vi "GUI_HPD_CCD.vi"() -> ()   [LabVIEW 2013]
uses:
  shared programs/GUI_Template/GUI_master/tcp_new_data_event.ctl
  shared programs/GUI_Template/GUI_master/tcp new data cluster.ctl
  <vilib>/vision/Image Controls.llb/IMAQ Image.ctl
panel:
  out "image::3":T1(plugin-control) caption="image"
  out "GUIdevice 3":string="HPD_CCD"
  in  "exposure::2":dbl=0.001 caption="exposure" min=0.0001 max=1.0 format="%_4p"
  in  "GUIdevice 2":string="HPD_CCD"
  out "image::2":T1(plugin-control) caption="image"
  out "tcp data event":T2
  in  "Refresh Button":bool
  in  "Select device":string(combo)="FrogHPD"
  in  "stop":bool
  in  "trigger::1":bool caption="Trigger"
  in  "gain::1":dbl=0.001 caption="gain" min=0.0 max=24.0 format="%_4f"
  in  "centroidy::1":dbl=0.001 caption="centroid y" min=0.0 max=0.0 format="%_4f"
  in  "centroidx::1":dbl=0.001 caption="centroid x" min=0.0 max=0.0 format="%_4f"
  in  "exposure::1":dbl=0.001 caption="exposure" min=0.0001 max=1.0 format="%_4p"
  out "image::1":T1(plugin-control) caption="image"
  out "GUIdevice 1":string="HPD_CCD"
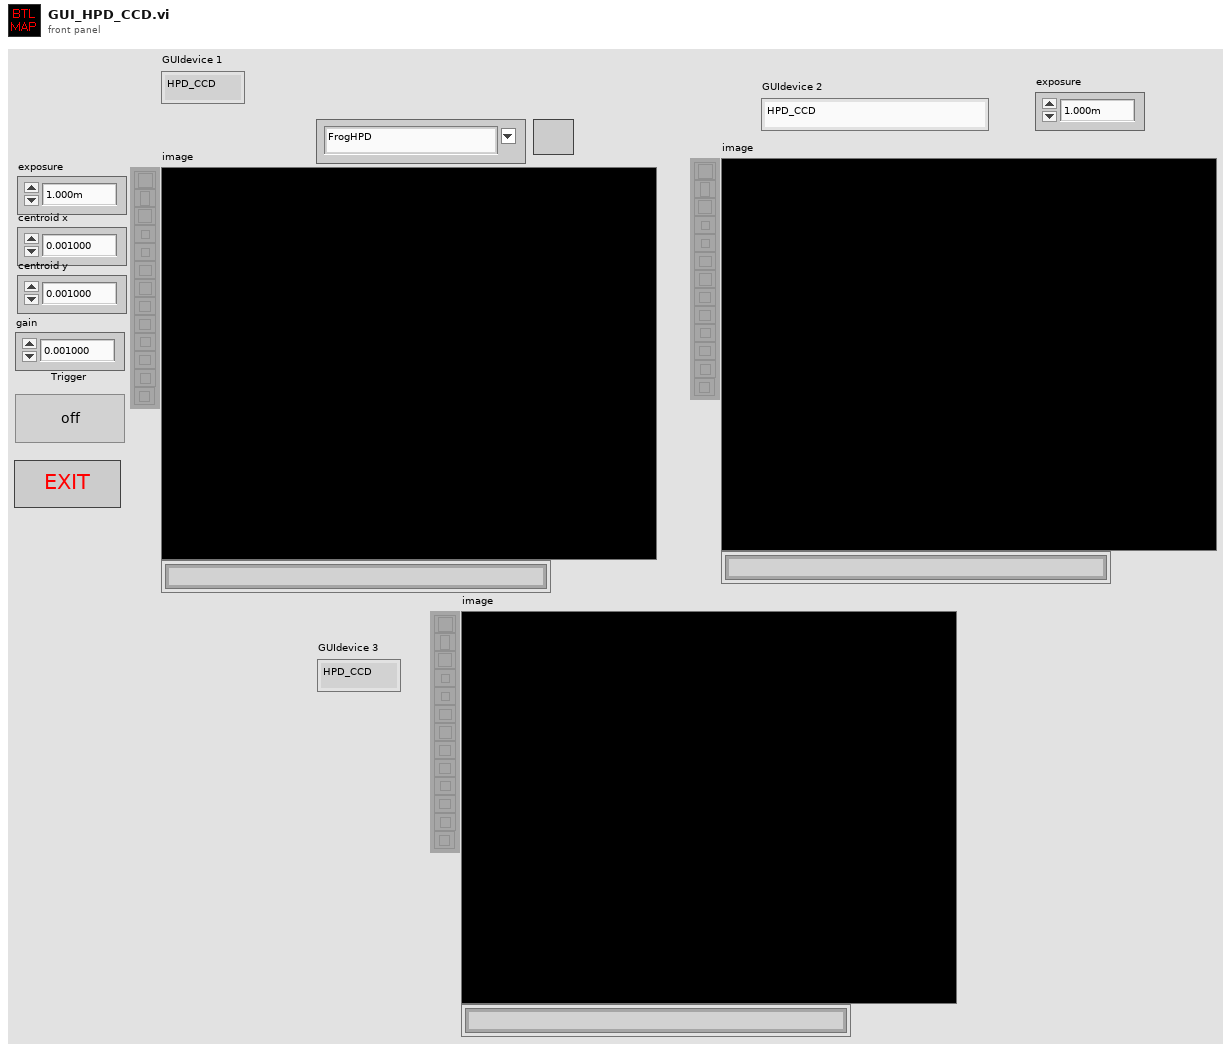
[diagram p1: front panel]
types:
  T1 = typedef "IMAQ Image.ctl" = refnum<image>
  T2 = typedef "tcp_new_data_event.ctl" = refnum<user-event>
  T3 = enum32{"invalid app kind", "Development System", "Run Time System", "Student Edition", "Embedded LabVIEW", "Evaluation", "Custom"}
  T4 = typedef "tcp new data cluster.ctl" = cluster{"EventEnum":enum16{"new data", "connection status update"}, "Device name":string}
  T5 = enum32{"Invalid", "Standard", "Closed", "Hidden", "Minimized", "Maximized"}
  T6 = cluster{"Core":cluster{"Current VI Reference":refnum<vi>, "Close Panel on Exit?":bool}, "Your Boolean data":bool, "Your string data":string, "SuperGUI":cluster{"STOP queue":refnum<queue>, "SuperGUI ref":refnum<vi>}}
  T7 = cluster{"STOP queue":refnum<queue>, "SuperGUI ref":refnum<vi>}
  T8 = cluster{"Current VI Reference":refnum<vi>, "Close Panel on Exit?":bool}
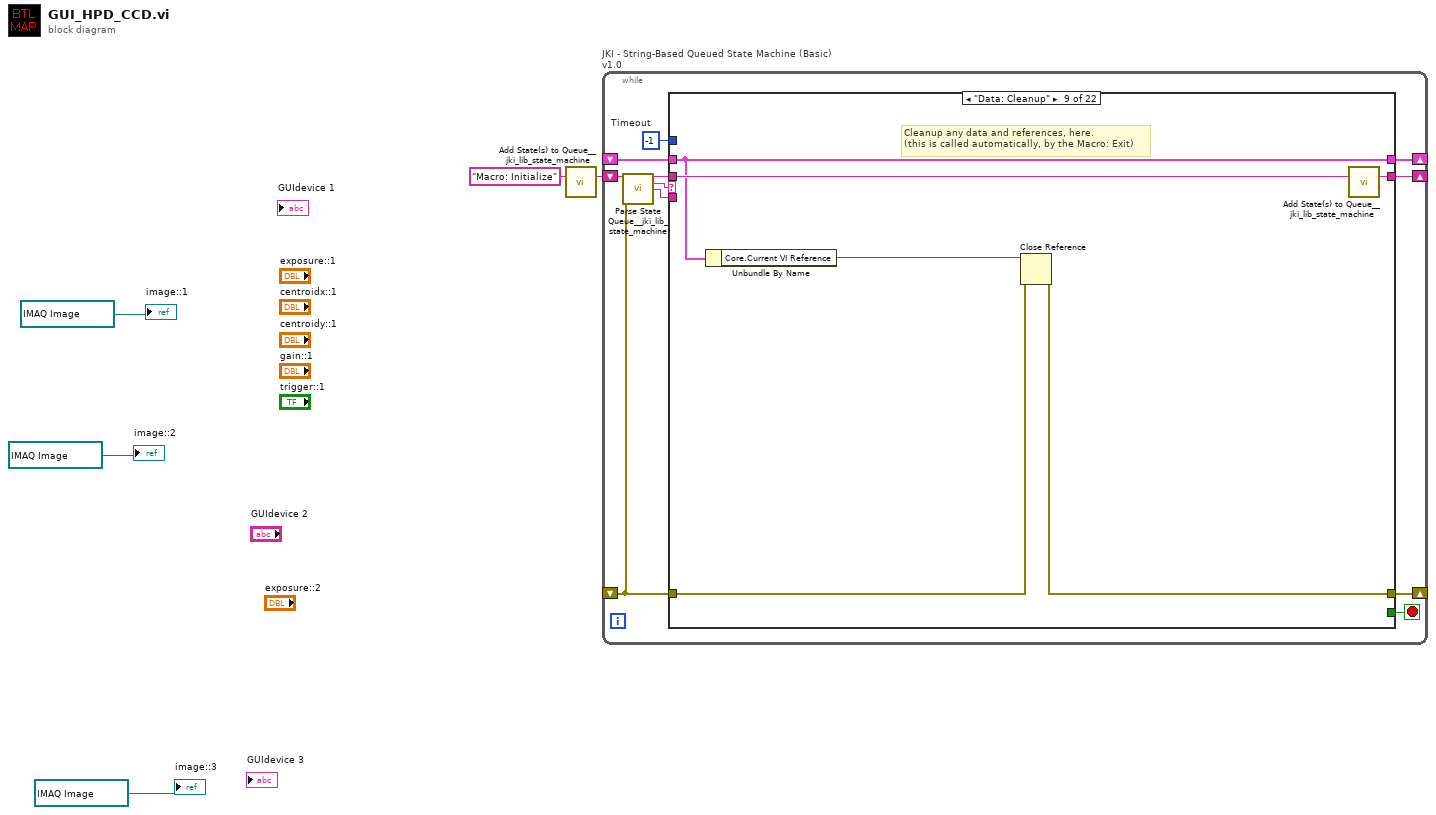
[diagram p0: block diagram]
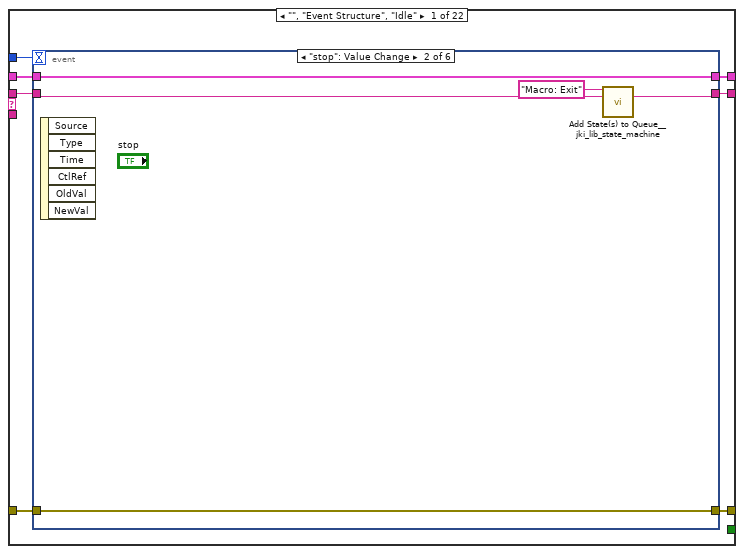
[diagram p2: hidden frame]
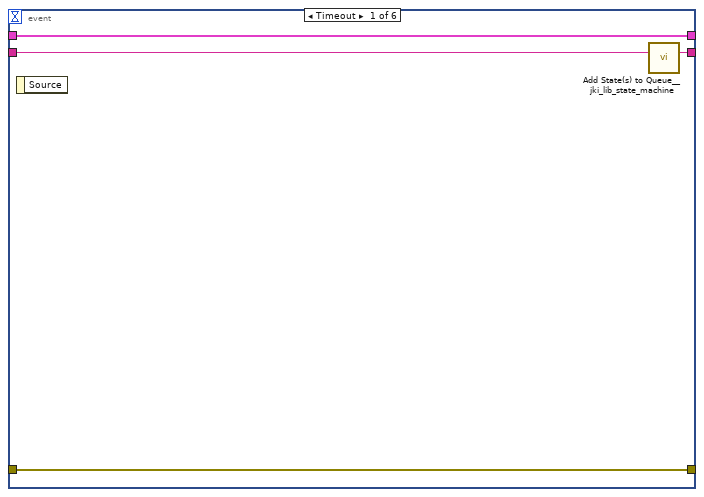
[diagram p3: hidden frame]
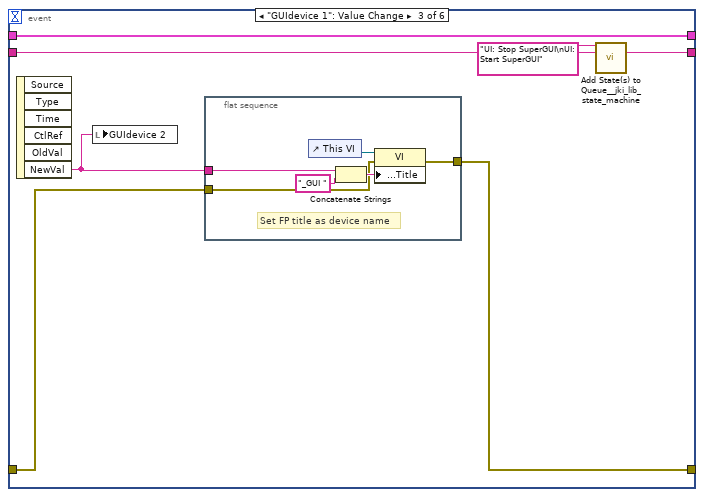
[diagram p4: hidden frame]
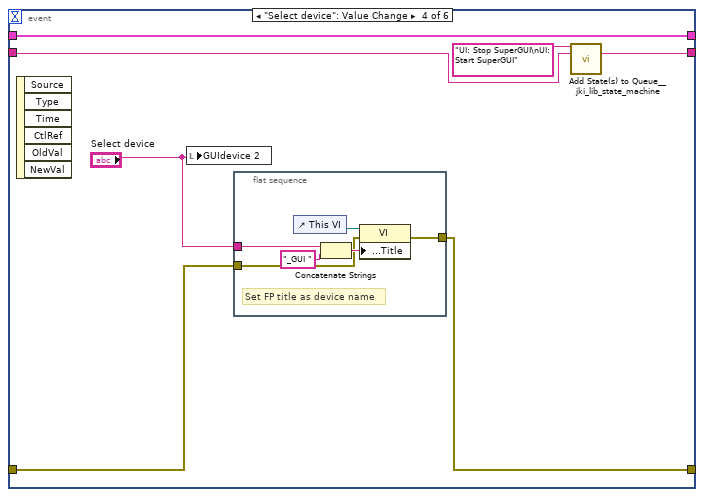
[diagram p5: hidden frame]
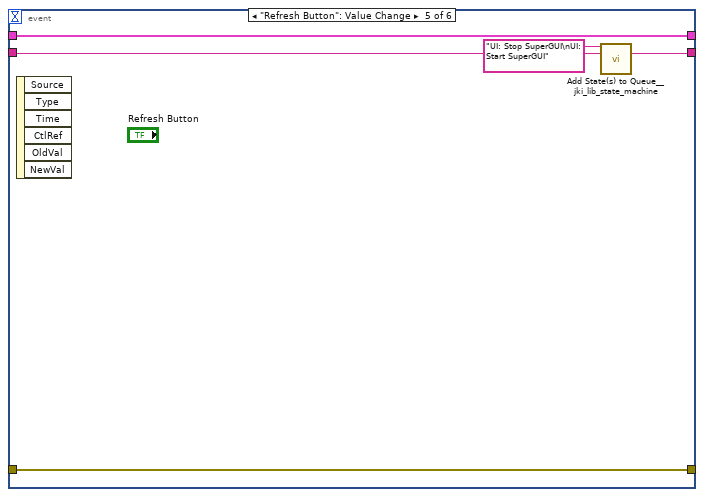
[diagram p6: hidden frame]
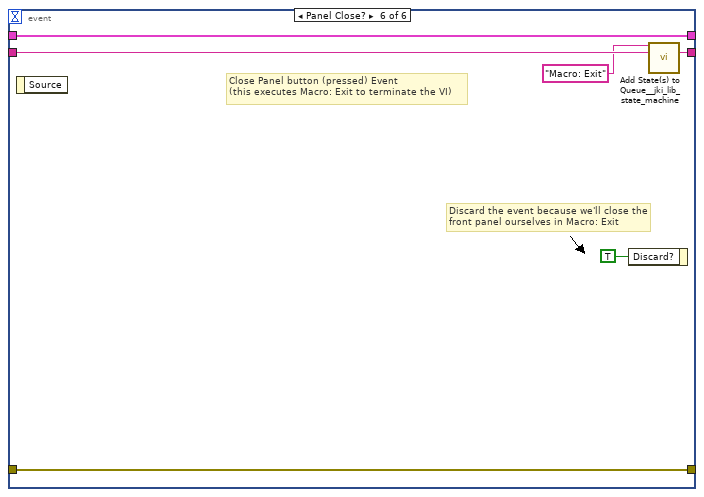
[diagram p7: hidden frame]
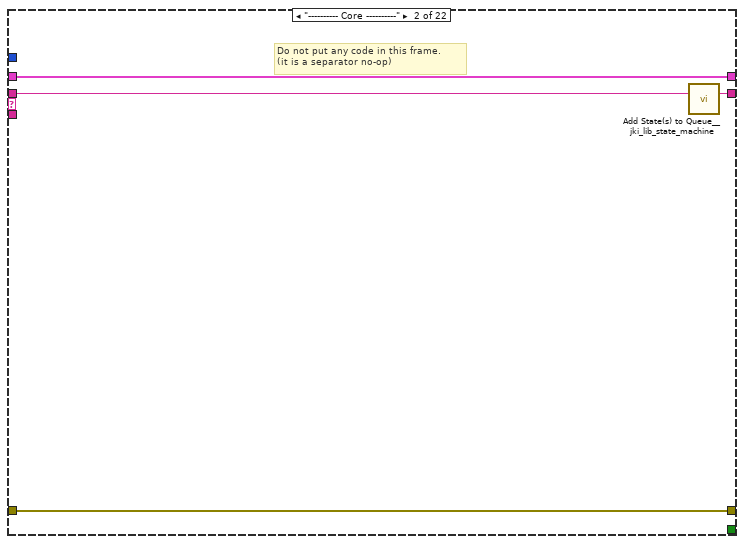
[diagram p8: hidden frame]
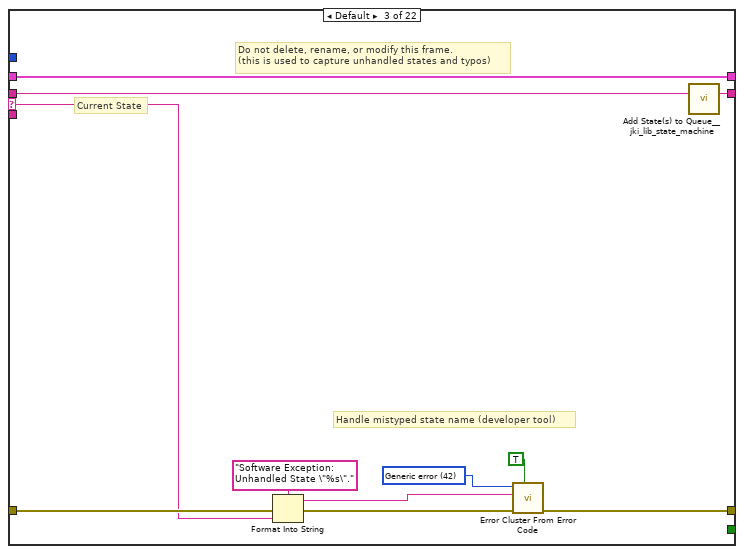
[diagram p9: hidden frame]
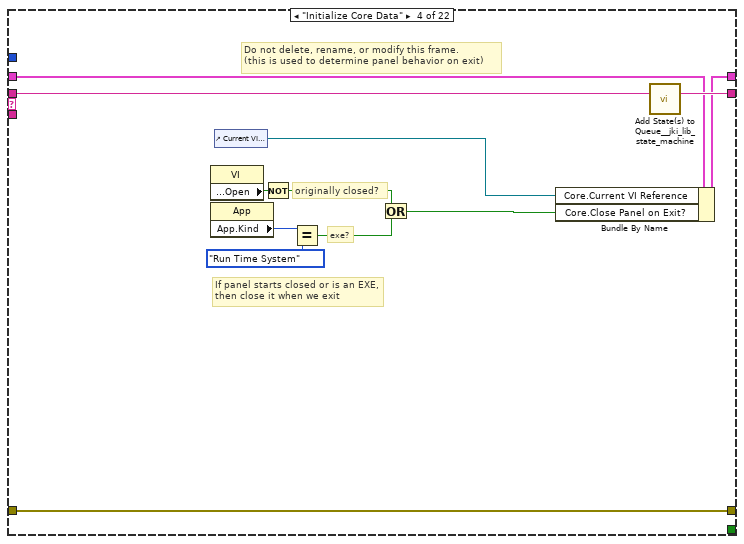
[diagram p10: hidden frame]
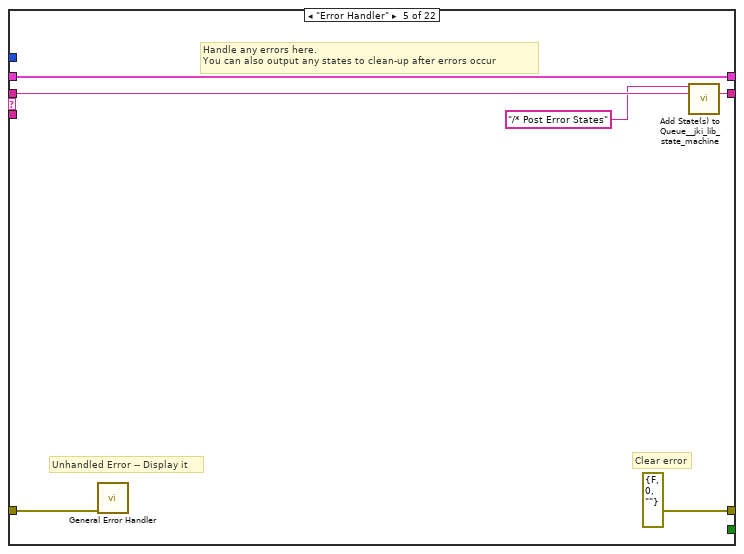
[diagram p11: hidden frame]
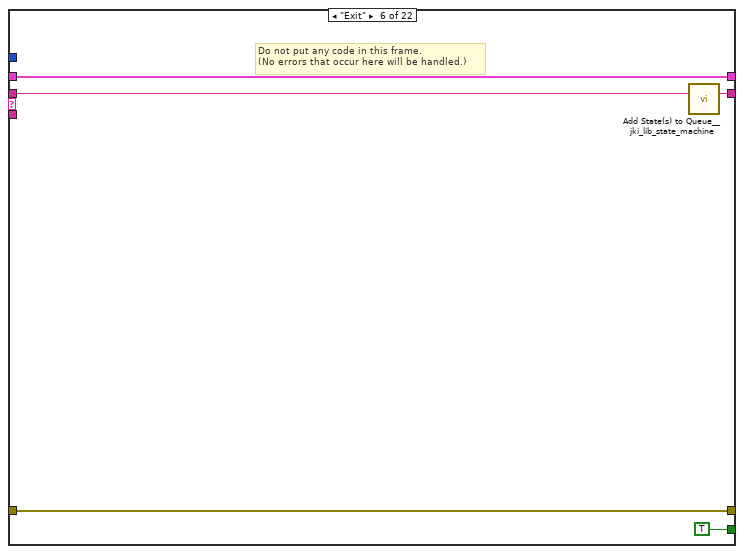
[diagram p12: hidden frame]
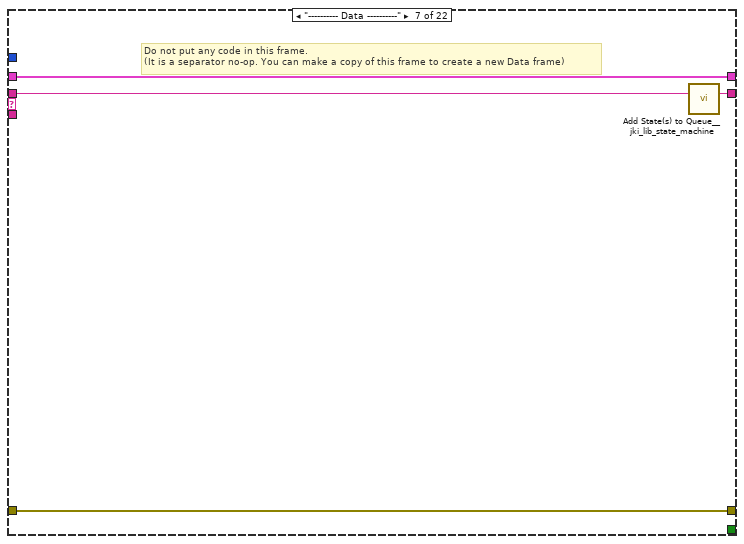
[diagram p13: hidden frame]
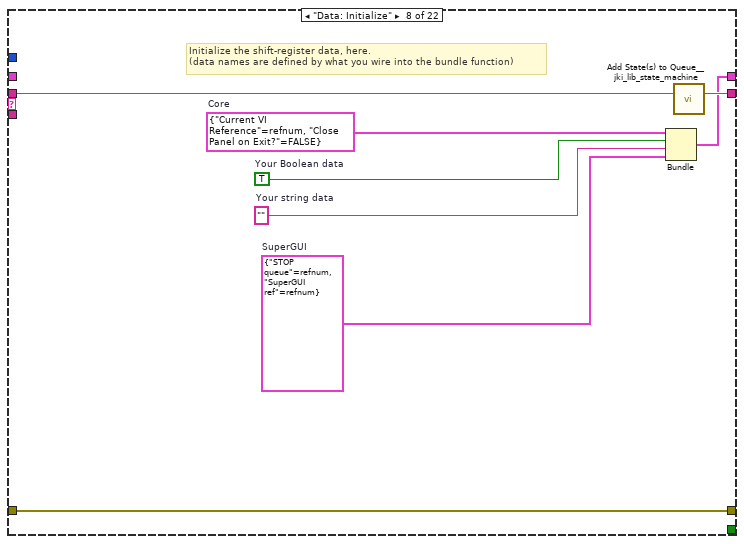
[diagram p14: hidden frame]
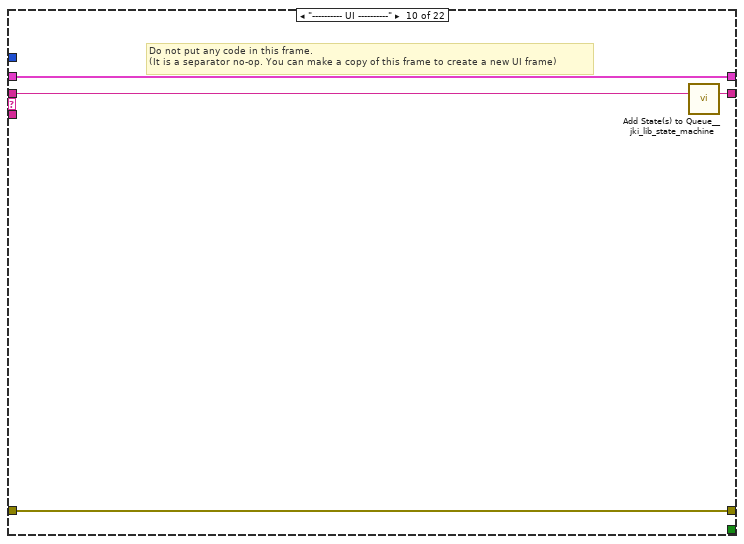
[diagram p15: hidden frame]
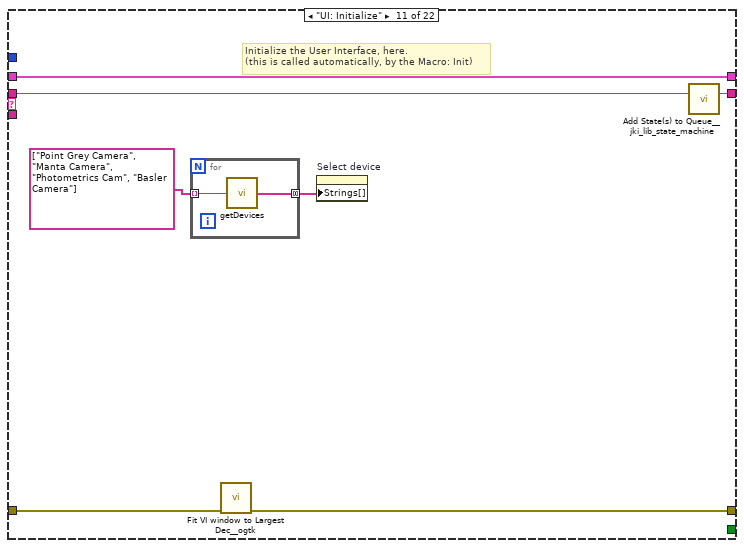
[diagram p16: hidden frame]
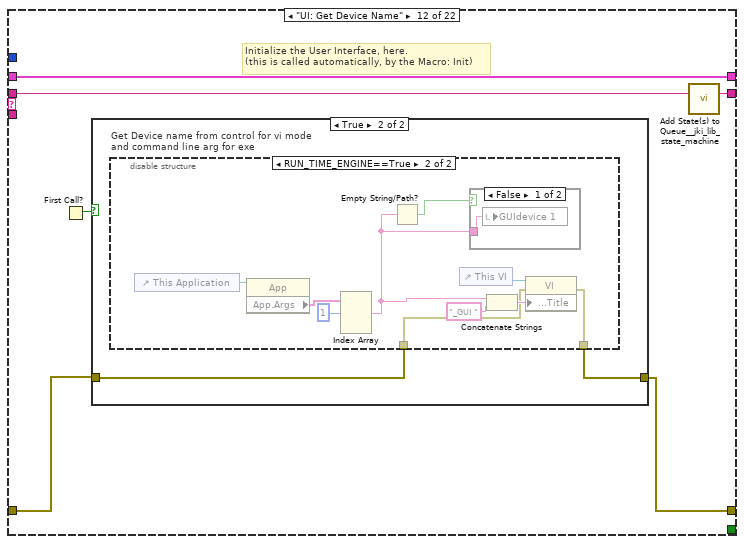
[diagram p17: hidden frame]
diagram:
  n1 = call <vilib>:"Add State(s) to Queue__jki_lib_state_machine.vi"("State(s) in (\"\")"="Macro: Initialize") -> ("States Out"=w4:string)  [unwired: 14 in]
  n2 = while "JKI - String-Based Queued State Machine (Basic) v1.0" {
    shift-right: [w9] -> _
    shift-left: _ -> [w8]
    shift-right: [w12] -> _
    shift-left: _ -> [w6]
    shift-right: [w11] -> _
    shift-left: w4 -> [w13]
    stop <- w10 stop-if-true
    w7 = -1  # Timeout
    n3 = call <vilib>:"Parse State Queue__jki_lib_state_machine.vi"("State Queue"=w13, "Error In (no error)"=w6) -> ("Remaining States"=w15:string, "Current State"=w16:string, "Arguments"=w14:string)  [unwired: 11 in]
    n4 = case shown="\"Data: Cleanup\"" w16 {
      selector: w16 -> [_ _ w74 _ _ _ _ _ _ _ _ _ _ _ _ _ _ _ _ _ _ _]
      tunnel: w15 -> [w23 w73 w78 w96 w102 w107 w111 w119 w125 w129 w136 w144 w179 w187 w193 w204 w230 w235 w245 w249 w253 w257]
      tunnel: w14 -> [_ _ _ _ _ _ _ _ _ _ _ _ _ _ w188 w198 _ _ _ _ _ _]
      tunnel: w8 -> [w21 w70 w76 w87 w99 w105 w108 _ w120 w126 w134 w142 w170 w182 w191 w200 w227 w232 w242 w246 w250 w254]
      tunnel: [w20 w71 w80 w93 errorcluster {"status"=FALSE, "code"=0, "source"=""} ("error out") w104 w109 w116 w121 w127 w132 w139 w163 w180 w189 w201 w228 w233 w243 w247 w251 w255] -> w12
      tunnel: w6 -> [w19 w71 w79 w93 w98 w104 w109 w116 w122 w127 w133 w140 w164 w181 w190 w202 w228 w233 w243 w247 w251 w255]
      tunnel: [w22 w72 w77 w95 w101 w106 w110 w118 w124 w128 w135 w143 w178 w186 w192 w203 w229 w234 w244 w248 w252 w256] -> w11
      tunnel: [_ _ _ _ _ TRUE _ _ _ _ _ _ _ _ _ _ _ _ _ _ _ _] -> w10
      tunnel: [w18 w70 w76 w94 w99 w105 w108 w117 w120 w126 w134 w142 w169 w182 w191 w200 w227 w232 w242 w246 w250 w254] -> w9
      tunnel: w7 -> [w17 _ _ _ _ _ _ _ _ _ _ _ _ _ _ _ _ _ _ _ _ _]
      frame "", "Event Structure", "Idle" {
        n5 = event shown="[1] \"stop\": Value Change" {
          selector: _ -> [_ _ _ _ _ _]
          dyn-events: _ -> [_ _ _ _ _ _]
          timeout: w17 -> [_ _ _ _ _ _]
          tunnel: w23 -> [w27 w30 w36 w48 w61 w69]
          tunnel: [w26 w29 w35 w47 w60 w68] -> w22
          tunnel: w21 -> [w24 w32 w39 w52 w63 w66]
          tunnel: [w25 w31 w37 w50 w62 w67] -> w20
          tunnel: w19 -> [w25 w31 w38 w51 w62 w67]
          tunnel: [w24 w32 w39 w52 w63 w66] -> w18
          event Timeout {
            n6 = event-data() -> ()  [unwired: 1 in, 1 out]
            n7 = call <vilib>:"Add State(s) to Queue__jki_lib_state_machine.vi"("State(s) in (\"\")"=w27) -> ("States Out"=w26:string)  [unwired: 14 in]
          }
          event "stop": Value Change {
            n8 = event-data() -> ()  [unwired: 1 in, 6 out]
            n9 = call <vilib>:"Add State(s) to Queue__jki_lib_state_machine.vi"("State(s) in Front (\"\")"="Macro: Exit", "State(s) in (\"\")"=w30) -> ("States Out"=w29:string)  [unwired: 13 in]
          }
          event "GUIdevice 1": Value Change {
            n10 = event-data() -> ("NewVal"=w33:string)  [unwired: 1 in, 5 out]
            n11 = local write "GUIdevice 2"(w33) -> ()
            n12 = flat-sequence {
              tunnel: [w42] -> w37
              tunnel: w38 -> [w41]
              tunnel: w33 -> [w40]
              frame #0 {
                # "Set FP title as device name"
                n13 = control-ref of="This VI"() -> (w45:refnum<vi>)
                n14 = Concatenate Strings(w40, "_GUI ") -> (w44:string)
                n15 = property class="VI"(reference=w45, error in=w41, "Front Panel.Title"=w44) -> (error out=w42:errorcluster)  [unwired: 1 out]
              }
            }
            n16 = call <vilib>:"Add State(s) to Queue__jki_lib_state_machine.vi"("State(s) in Front (\"\")"="UI: Stop SuperGUI\nUI: Start SuperGUI", "State(s) in (\"\")"=w36) -> ("States Out"=w35:string)  [unwired: 13 in]
          }
          event "Select device": Value Change {
            n17 = event-data() -> ()  [unwired: 1 in, 6 out]
            n18 = local write "GUIdevice 2"("Select device") -> ()
            n19 = flat-sequence {
              tunnel: [w55] -> w50
              tunnel: w51 -> [w54]
              tunnel: "Select device" -> [w53]
              frame #0 {
                # "Set FP title as device name"
                n20 = control-ref of="This VI"() -> (w58:refnum<vi>)
                n21 = Concatenate Strings(w53, "_GUI ") -> (w57:string)
                n22 = property class="VI"(reference=w58, error in=w54, "Front Panel.Title"=w57) -> (error out=w55:errorcluster)  [unwired: 1 out]
              }
            }
            n23 = call <vilib>:"Add State(s) to Queue__jki_lib_state_machine.vi"("State(s) in Front (\"\")"="UI: Stop SuperGUI\nUI: Start SuperGUI", "State(s) in (\"\")"=w48) -> ("States Out"=w47:string)  [unwired: 13 in]
          }
          event "Refresh Button": Value Change {
            n24 = event-data() -> ()  [unwired: 1 in, 6 out]
            n25 = call <vilib>:"Add State(s) to Queue__jki_lib_state_machine.vi"("State(s) in Front (\"\")"="UI: Stop SuperGUI\nUI: Start SuperGUI", "State(s) in (\"\")"=w61) -> ("States Out"=w60:string)  [unwired: 13 in]
          }
          event Panel Close? {
            # "Discard the event because we'll close the front panel ourselves in Macro: Exit"
            # "Close Panel button (pressed) Event\n(this executes Macro: Exit to terminate the VI)"
            n26 = event-data() -> ()  [unwired: 1 in, 1 out]
            n27 = event-data("Discard?"=TRUE) -> ()  [unwired: 1 in, 1 out]
            n28 = call <vilib>:"Add State(s) to Queue__jki_lib_state_machine.vi"("State(s) in Front (\"\")"="Macro: Exit", "State(s) in (\"\")"=w69) -> ("States Out"=w68:string)  [unwired: 13 in]
          }
        }
      }
      frame "---------- Core ----------" {
        # "Do not put any code in this frame.\n(it is a separator no-op)"
        n29 = call <vilib>:"Add State(s) to Queue__jki_lib_state_machine.vi"("State(s) in (\"\")"=w73) -> ("States Out"=w72:string)  [unwired: 14 in]
      }
      frame Default {
        w83 = 42 items=["No error", "Argument error", "Memory is full", "Out of zone", "End of file", "File already open", "Generic file I/O error", "File not found", "File permission error", "Disk is full", "Duplicate path", "Too many files open", "System feature not enabled", "Resource file not found", "Cannot add resource", "Resource not found", "Image not found", "Image memory error", "Pen does not exist", "Config type invalid", "Config token not found", "Config parse error", "Config memory error", "Bad external code format", "Bad external code offset", "External code not present", "Null window", "Destroy window error", "Null menu", "Print aborted", "Bad print record", "Print driver error", "Windows error during printing", "Memory error during printing", "Print dialog error", "Generic print error", "Invalid device refnum", "Device not found", "Device parameter error", "Device unit error", "Cannot open device", "Device call aborted", "Generic error", "Cancelled by user", "Object ID too low", "Object ID too high", "Object not in heap", "Unknown heap", "Unknown object (invalid DefProc)", "Unknown object (DefProc not in table)", "Message out of range", "Invalid (null) method", "Unknown message", "Manager call not supported", "Bad address", "Network operation in progress", "Network operation timed out", "Connection is busy", "Network attribute not supported", "Network error", "Address in use", "System out of memory", "Connection aborted", "Connection refused", "Not connected", "Already connected", "Connection closed", "Initialization error (interapplication manager)", "Bad occurrence", "Wait on unbound occurrence handler", "Occurrence queue overflow", "Datalog type conflict", "Unused", "Unrecognized type (interapplication manager)", "Memory corrupt", "Failed to make temporary DLL", "Old CIN version", "Drag socket not found", "Failed to load drop-object", "Failed to register OLE object", "Failed to release OLE object", "Format specifier type mismatch", "Unknown format specifier", "Too few format specifiers", "Too many format specifiers", "Scan failed", "Newer CIN version", "Error converting to variant", "Runtime menu error", "Password tampered", "Variant attribute not found", "Incompatible variant data type", "Event data is not available", "Event Store is not present", "Occurrence is not found", "Event Queue is not created", "Event info is not available", "Refnum passed is NULL", "Error retrieving Class GUID", "Error retrieving CoClass GUID", "Error retrieving TypeLib GUID.", "Bad built application magic bytes.", "Specific driver is different from the specific driver associated with the Logical Name.", "There is no session opened to the class driver.", "Max Error", "MAX - Error with config objects", "MAX - Error loading configuration", "MAX - Group not supported"]
        # "Current State"
        # "Do not delete, rename, or modify this frame.\n(this is used to capture unhandled states and typos)"
        # "Handle mistyped state name (developer tool)"
        n30 = Format Into String(format string="Software Exception: Unhandled State \"%s\"." ("message"), error in=w79, w74) -> (resulting string=w82:string, error out=w81:errorcluster)  [unwired: 1 in]
        n31 = call <vilib>:"Error Cluster From Error Code.vi"("show call chain? (False)"=TRUE, "error in (no error)"=w81, "error message (\"\")"=w82, "error code (0)"=w83) -> ("error out"=w80:errorcluster)  [unwired: 5 in]
        n32 = call <vilib>:"Add State(s) to Queue__jki_lib_state_machine.vi"("State(s) in (\"\")"=w78) -> ("States Out"=w77:string)  [unwired: 14 in]
      }
      frame "Initialize Core Data" {
        # "Do not delete, rename, or modify this frame.\n(this is used to determine panel behavior on exit)"
        # "originally closed?"
        # "exe?"
        # "If panel starts closed or is an EXE, then close it when we exit"
        n33 = property class="VI"() -> ("Front Panel.Open"=w92:bool)  [unwired: 2 in, 2 out]
        n34 = property class="App"() -> ("App.Kind"=w91:T3)  [unwired: 2 in, 2 out]
        n35 = control-ref of="Current VI Reference"() -> (w85:refnum<vi>)
        n36 = Not(x=w92) -> (.not. x?=w89:bool)
        n37 = Equal?(x=w91, y=T3."Run Time System" ("Application:Kind")) -> (x = y?=w88:bool)
        n38 = Or(x=w89, y=w88) -> (x .or. y?=w86:bool)
        n39 = Bundle By Name(cluster=w87, "Core.Current VI Reference"=w85, "Core.Close Panel on Exit?"=w86) -> (w94:T6)
        n40 = call <vilib>:"Add State(s) to Queue__jki_lib_state_machine.vi"("State(s) in (\"\")"=w96) -> ("States Out"=w95:string)  [unwired: 14 in]
      }
      frame "Error Handler" {
        # "Unhandled Error -- Display it"
        # "Handle any errors here.\nYou can also output any states to clean-up after errors occur"
        # "Clear error"
        n41 = call <vilib>:"General Error Handler.vi"("error in (no error)"=w98) -> ()  [unwired: 10 in, 5 out]
        n42 = call <vilib>:"Add State(s) to Queue__jki_lib_state_machine.vi"("State(s) in Front (\"\")"="/* Post Error States", "State(s) in (\"\")"=w102) -> ("States Out"=w101:string)  [unwired: 13 in]
      }
      frame "Exit" {
        # "Do not put any code in this frame.\n(No errors that occur here will be handled.)"
        n43 = call <vilib>:"Add State(s) to Queue__jki_lib_state_machine.vi"("State(s) in (\"\")"=w107) -> ("States Out"=w106:string)  [unwired: 14 in]
      }
      frame "---------- Data ----------" {
        # "Do not put any code in this frame.\n(It is a separator no-op. You can make a copy of this frame to create a new Data frame)"
        n44 = call <vilib>:"Add State(s) to Queue__jki_lib_state_machine.vi"("State(s) in (\"\")"=w111) -> ("States Out"=w110:string)  [unwired: 14 in]
      }
      frame "Data: Initialize" {
        w112 = T7 {"STOP queue"=refnum, "SuperGUI ref"=refnum}  # SuperGUI
        w113 = T8 {"Current VI Reference"=refnum, "Close Panel on Exit?"=FALSE}  # Core
        w115 = TRUE  # Your Boolean data
        w114 = ""  # Your string data
        # "Initialize the shift-register data, here.\n(data names are defined by what you wire into the bundle function)"
        n45 = Bundle("Core"=w113, "Your Boolean data"=w115, "Your string data"=w114, "SuperGUI"=w112) -> (w117:T6)  [unwired: 1 in]
        n46 = call <vilib>:"Add State(s) to Queue__jki_lib_state_machine.vi"("State(s) in (\"\")"=w119) -> ("States Out"=w118:string)  [unwired: 14 in]
      }
      frame "Data: Cleanup" {
        # "Cleanup any data and references, here.\n(this is called automatically, by the Macro: Exit)"
        n47 = Unbundle By Name(w120) -> ("Core.Current VI Reference"=w123:refnum<vi>)
        n48 = Close Reference(reference=w123, error in (no error)=w122) -> (error out=w121:errorcluster)
        n49 = call <vilib>:"Add State(s) to Queue__jki_lib_state_machine.vi"("State(s) in (\"\")"=w125) -> ("States Out"=w124:string)  [unwired: 14 in]
      }
      frame "---------- UI ----------" {
        # "Do not put any code in this frame.\n(It is a separator no-op. You can make a copy of this frame to create a new UI frame)"
        n50 = call <vilib>:"Add State(s) to Queue__jki_lib_state_machine.vi"("State(s) in (\"\")"=w129) -> ("States Out"=w128:string)  [unwired: 14 in]
      }
      frame "UI: Initialize" {
        # "Initialize the User Interface, here.\n(this is called automatically, by the Macro: Init)"
        n51 = for {
          tunnel: string[] ["Point Grey Camera", "Manta Camera", "Photometrics Cam", "Basler Camera"] -> [w138] mode=indexing
          tunnel: [w137] -> w130 mode=concatenating
          n52 = call "getDevices.vi"("Device Class"=w138) -> ("All Devices"=w137:string[])
        }
        n53 = call <userlib>:"Fit VI window to Largest Dec__ogtk.vi"("error in (no error)"=w133) -> ("error out"=w132:errorcluster)  [unwired: 5 in, 1 out]
        n54 = property on="Select device" class="CmbBox"("Strings[]"=w130) -> ()  [unwired: 2 in, 2 out]
        n55 = call <vilib>:"Add State(s) to Queue__jki_lib_state_machine.vi"("State(s) in (\"\")"=w136) -> ("States Out"=w135:string)  [unwired: 14 in]
      }
      frame "UI: Get Device Name" {
        # "Initialize the User Interface, here.\n(this is called automatically, by the Macro: Init)"
        n56 = First Call?() -> (First Call?: T/F=w141:bool)
        n57 = case shown="True" w141 {
          tunnel: w140 -> [w145 w147]
          tunnel: [w145 w146] -> w139
          frame False {
          }
          frame True {
            n58 = disable-structure "Get Device name from control for vi mode\nand command line arg for exe" shown="RUN_TIME_ENGINE==True" {
              disable-tunnel: w147 -> [w148 w150]
              disable-tunnel: [w148 w149] -> w146
              frame condition #0 (active) {
              }
              frame condition #1 {
                n59 = control-ref of="This Application"() -> (w158:refnum<vi>)
                n60 = property class="App"(reference=w158) -> ("App.Args"=w157:string[])  [unwired: 1 in, 2 out]
                n61 = Index Array(array=w157, index #1=1 ("index")) -> (element #1=w151:string)  [unwired: 2 in, 2 out]
                n62 = Empty String/Path?(string/path=w151) -> (empty?=w155:bool)
                n63 = control-ref of="This VI"() -> (w154:refnum<vi>)
                n64 = case shown="False" w155 {
                  tunnel: w151 -> [w159 _]
                  frame False {
                    n65 = local write "GUIdevice 1"(w159) -> ()
                  }
                  frame True {
                  }
                }
                n66 = Concatenate Strings(w151, "_GUI ") -> (w153:string)
                n67 = property class="VI"(reference=w154, error in=w150, "Front Panel.Title"=w153) -> (error out=w149:errorcluster)  [unwired: 1 out]
              }
            }
          }
        }
        n68 = call <vilib>:"Add State(s) to Queue__jki_lib_state_machine.vi"("State(s) in (\"\")"=w144) -> ("States Out"=w143:string)  [unwired: 14 in]
      }
      frame "UI: Start SuperGUI" {
        # "create stop queue for supergui and its clones"
        # "x100 abort will be dependent on caller VI\nx80 abort will be independent of caller vi, this will abort vi when labview is closed."
        # "Start SuperGUI asynchronous way"
        n69 = vi-ref "GUI_Master_subvi_reentrant_queues.vi"() -> (w162:refnum<vi>)
        n70 = property class="VI"(reference=w162) -> ("Path"=w161:path)  [unwired: 1 in, 2 out]
        n71 = Create User Event(user event datatype=T4 {"EventEnum"=enum."new data", "Device name"="Device name"} ("New Event"), error in=w164) -> (user event=w165:refnum<user-event>, error out=w171:errorcluster)
        "tcp data event" <- w165
        n72 = control-ref of="This Application"() -> (w168:refnum<vi>)
        n73 = control-ref of="This VI"() -> (w167:refnum<vi>)
        n74 = Open VI Reference(type specifier VI Refnum (for type only)=refnum<vi> refnum, vi path=w161, options=256) -> (vi reference=w177:refnum<vi>, error out=w176:errorcluster)  [unwired: 3 in]
        n75 = register-events(w165) -> ()  [unwired: 2 in, 2 out]
        n76 = call "supergui create stop queue.vi"() -> ("STOP Queue out"=w173:refnum<queue>)  [unwired: 11 in]
        n77 = Current VI's Menubar() -> (w166:refnum<k9>)
        n78 = call-by-ref "Start Asynchronous Call"(reference=w177, error in=w176, "STOP Queue in"=w173, "This Application"=w168, 8:"error in (no error)"=w171, "tcp data event"=w165, "Caller menu reference"=w166, "Caller VI ref"=w167) -> (reference out=w160:refnum<vi>, error out=w163:errorcluster)  [unwired: 5 in, 1 out]
        n79 = Bundle By Name(cluster=w170, "SuperGUI.SuperGUI ref"=w160, "SuperGUI.STOP queue"=w173) -> (w169:T6)
        n80 = call <vilib>:"Add State(s) to Queue__jki_lib_state_machine.vi"("State(s) in (\"\")"=w179) -> ("States Out"=w178:string)  [unwired: 14 in]
      }
      frame "UI: Stop SuperGUI" {
        # "Stop Supergui Clone and wait until it exit properly"
        n81 = Unbundle By Name(w182) -> ("SuperGUI.SuperGUI ref"=w184:refnum<vi>, "SuperGUI.STOP queue"=w183:refnum<queue>)
        n82 = Release Queue(queue=w183, error in (no error)=w181) -> (error out=w185:errorcluster)  [unwired: 1 in, 2 out]
        n83 = call-by-ref "Wait On Asynchronous Call"(reference=w184, error in=w185) -> ("error out"=w180:errorcluster)  [unwired: 11 in, 2 out]
        n84 = call <vilib>:"Add State(s) to Queue__jki_lib_state_machine.vi"("State(s) in (\"\")"=w187) -> ("States Out"=w186:string)  [unwired: 14 in]
      }
      frame "UI: Cursor Set" {
        # "Argument"
        # "Set and Unset Cursor Busy.\n(Usage: \"UI: Cursor Set >> Busy|Idle\")"
        n85 = case shown="\"Idle\", Default" w188 {
          tunnel: w190 -> [w195 w197]
          tunnel: [w194 w196] -> w189
          frame "Idle", Default {
            n86 = call <vilib>:"Unset Busy.vi"("error in (no error)"=w195) -> ("error out"=w194:errorcluster)  [unwired: 10 in]
          }
          frame "Busy" {
            n87 = call <vilib>:"Set Busy.vi"("error in (no error)"=w197) -> ("error out"=w196:errorcluster)  [unwired: 9 in, 1 out]
          }
        }
        n88 = call <vilib>:"Add State(s) to Queue__jki_lib_state_machine.vi"("State(s) in (\"\")"=w193) -> ("States Out"=w192:string)  [unwired: 14 in]
      }
      frame "UI: Front Panel State" {
        # "Argument"
        # "Set Front Panel Open or Closed\n(Usage: \"UI: Front Panel State >> Open|Close\")"
        n89 = Unbundle By Name(w200) -> ("Core.Current VI Reference"=w199:refnum<vi>)
        n90 = case shown="\"Open\", Default" w198 {
          tunnel: w202 -> [w208 w221]
          tunnel: [w210 w222] -> w201
          tunnel: w199 -> [w209 w219]
          frame "Open", Default {
            n91 = property class="VI"(reference=w209, error in=w208) -> (reference out=w206:refnum<vi>, error out=w207:errorcluster, "Front Panel.Open"=w205:bool)
            n92 = case shown="False" w205 {
              tunnel: [w213 w216] -> w210
              tunnel: w207 -> [w212 w216]
              tunnel: w206 -> [w211 _]
              frame False {
                n93 = invoke class="VI" method="FP.Open"(reference=w211, error in=w212, "Activate"=TRUE, "State"=T5."Standard") -> (error out=w213:errorcluster)  [unwired: 1 in, 4 out]
              }
              frame True {
              }
            }
          }
          frame "Close" {
            n94 = property class="VI"(reference=w219, error in=w221) -> (reference out=w218:refnum<vi>, error out=w220:errorcluster, "Front Panel.Open"=w217:bool)
            n95 = case shown="True" w217 {
              tunnel: [w223 w226] -> w222
              tunnel: w220 -> [w223 w225]
              tunnel: w218 -> [_ w224]
              frame False {
              }
              frame True {
                n96 = invoke class="VI" method="FP.Close"(reference=w224, error in=w225) -> (error out=w226:errorcluster)  [unwired: 1 in, 2 out]
              }
            }
          }
        }
        n97 = call <vilib>:"Add State(s) to Queue__jki_lib_state_machine.vi"("State(s) in (\"\")"=w204) -> ("States Out"=w203:string)  [unwired: 14 in]
      }
      frame "---------- Macro ----------" {
        # "Do not put any code in this frame.\n(It is a separator no-op. You can make a copy of this frame to create a new Macro frame)"
        n98 = call <vilib>:"Add State(s) to Queue__jki_lib_state_machine.vi"("State(s) in (\"\")"=w230) -> ("States Out"=w229:string)  [unwired: 14 in]
      }
      frame "Macro: Initialize" {
        # "Initialization Macro\n(This is called once, when the VI starts)"
        n99 = call <vilib>:"Add State(s) to Queue__jki_lib_state_machine.vi"("State(s) in Front (\"\")"="Data: Initialize\nInitialize Core Data\nUI: Initialize\nUI: Get Device Name\nUI: Start SuperGUI\nUI: Front Panel State >> Open", "State(s) in (\"\")"=w235) -> ("States Out"=w234:string)  [unwired: 13 in]
      }
      frame "Macro: Exit" {
        # "Exit Macro\n(This is called once, when the VI exits)"
        n100 = Unbundle By Name(w242) -> ("Core.Close Panel on Exit?"=w241:bool)
        n101 = Select(t="UI: Front Panel State >> Close", s=w241, f="") -> (s? t:f=w238:string)
        n102 = call <vilib>:"Add State(s) to Queue__jki_lib_state_machine.vi"("State(s) in (\"\")"=w238, "State(s) at Back (\"\")"="Data: Cleanup\nExit") -> ("States Out"=w236:string)  [unwired: 13 in]
        n103 = call <vilib>:"Add State(s) to Queue__jki_lib_state_machine.vi"("State(s) in Front (\"\")"=w236, "State(s) in (\"\")"=w245) -> ("States Out"=w244:string)  [unwired: 13 in]
      }
      frame "---------- New Category ----------" {
        # "Template Separator\n(You can make a copy of, or modify, this frame)"
        n104 = call <vilib>:"Add State(s) to Queue__jki_lib_state_machine.vi"("State(s) in (\"\")"=w249) -> ("States Out"=w248:string)  [unwired: 14 in]
      }
      frame "New Category: 1" {
        # "Your code here.\n(You can make a copy of, or modify, this frame)"
        n105 = call <vilib>:"Add State(s) to Queue__jki_lib_state_machine.vi"("State(s) in (\"\")"=w253) -> ("States Out"=w252:string)  [unwired: 14 in]
      }
      frame "New Category: 2" {
        # "Your code here.\n(You can make a copy of, or modify, this frame)"
        n106 = call <vilib>:"Add State(s) to Queue__jki_lib_state_machine.vi"("State(s) in (\"\")"=w257) -> ("States Out"=w256:string)  [unwired: 14 in]
      }
    }
  }
  "image::1" <- T1 refnum ("image::1")
  "image::2" <- T1 refnum ("image::1")
  "image::3" <- T1 refnum ("image::1")
